vi "Label Exclusions.vi"(8 "error in (no error)":errorcluster, 11 "Flex Msg in":refnum<class "Flex Msg.lvclass">) -> (0 "error out":errorcluster, 3 "Label Exclusions":string[](array[string]))   [LabVIEW 2020, in "Msg.lvlib" / "Flex Msg.lvclass"]
doc: "Get label exclusions for the private data handler."
uses:
  Flex Msg.lvclass
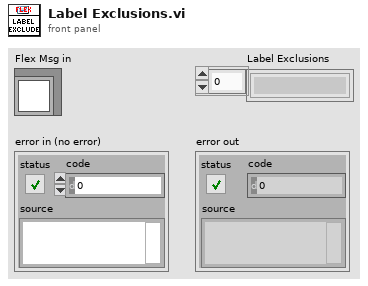
[diagram p1: front panel]
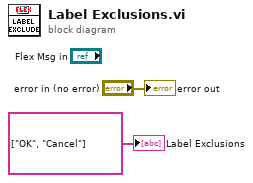
[diagram p0: block diagram]
diagram:
  "Label Exclusions" <- string[] ["OK", "Cancel"] ("Label Exclusions")
  "error out" <- "error in (no error)"
